vi "PassFailTest.vi"(4 "Sequence Context":T1) -> (0 "error out":errorcluster, 1 "Test Data":T2 {"Numeric Measurement" format="%.2f"})   [LabVIEW 2013]
doc: "Uses ActiveX to set the step result."
uses:
  <vilib>/addons/TestStand/_TSLegacy.llb/LabVIEW Test - Test Data.ctl
  <vilib>/addons/TestStand/_TSLegacy.llb/LabVIEW Test - Sequence Context.ctl
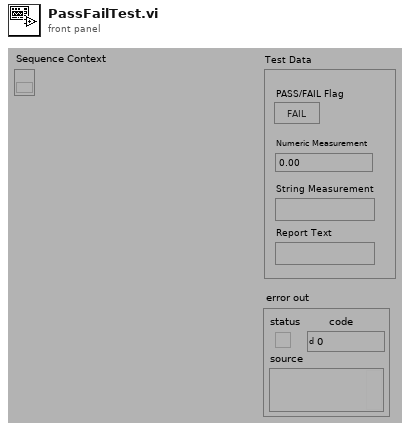
[diagram p1: front panel]
types:
  T1 = typedef "LabVIEW Test - Sequence Context.ctl" = refnum<k7>
  T2 = typedef "LabVIEW Test - Test Data.ctl" = cluster{"PASS/FAIL Flag":bool, "Numeric Measurement":dbl, "String Measurement":string, "Report Text":string}
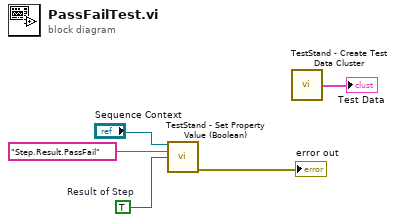
[diagram p0: block diagram]
diagram:
  w1 = TRUE  # Result of Step
  n1 = call <vilib>:"TestStand - Set Property Value (Boolean).vi"("Sequence Context In"="Sequence Context", "Lookup String"="Step.Result.PassFail", "New Value"=w1) -> ("error out"=→"error out":errorcluster)  [unwired: 2 in, 10 out]
  n2 = call <vilib>:"TestStand - Create Test Data Cluster.vi"() -> ("Test Data"=→"Test Data":T2)  [unwired: 4 in]
